vi "CatapultControl.vi"(10 "Fire Button":bool, 11 "ShooterDevRefIn":T1={"Wench Motor"={"DeviceStatus"={"status"=FALSE, "code"=0, "source"=""}, "Type"=enum."PWM", "PWM"={"Digital Module"=enum."Digital Module 1", "PWM Channel"=enum."Invalid", "DeadBand"={"Name"="", "maxPositivePwm"=0, "minPositivePwm"=0, "centerPwm"=0, "maxNegativePwm"=0, "minNegativePwm"=0, "angularRange"=0}}, "CAN"={"Device Number"=0, "Control Mode"=enum."Percent VBus", "Semaphore"=refnum, "Max Vout"=12.0}, "Invert"=FALSE, "TransformRef"=refnum, "InvTransformRef"=refnum}, "Lower Wench Limit"={"DevStatus"={"status"=FALSE, "code"=0, "source"=""}, "DIO Channel"=enum."DIO 1", "Digital Module"=enum."Digital Module 1"}, "Clutch Engaged Sensor"={"DevStatus"={"status"=FALSE, "code"=0, "source"=""}, "DIO Channel"=enum."DIO 1", "Digital Module"=enum."Digital Module 1"}, "Wench Encoder"={"DevStatus"={"status"=FALSE, "code"=0, "source"=""}, "EncoderIndex"=enum."Invalid", "CounterIndex"=enum."Invalid", "DistancePerCount"=1.0, "Decoding Type"=enum."4x"}, "Fire Sensor"={"DevStatus"={"status"=FALSE, "code"=0, "source"=""}, "DIO Channel"=enum."DIO 1", "Digital Module"=enum."Digital Module 1"}, "Worm Motor"={"DeviceStatus"={"status"=FALSE, "code"=0, "source"=""}, "Type"=enum."PWM", "PWM"={"Digital Module"=enum."Digital Module 1", "PWM Channel"=enum."Invalid", "DeadBand"={"Name"="", "maxPositivePwm"=0, "minPositivePwm"=0, "centerPwm"=0, "maxNegativePwm"=0, "minNegativePwm"=0, "angularRange"=0}}, "CAN"={"Device Number"=0, "Control Mode"=enum."Percent VBus", "Semaphore"=refnum, "Max Vout"=12.0}, "Invert"=FALSE, "TransformRef"=refnum, "InvTransformRef"=refnum}, "Minimum Worm Sensor"={"DevStatus"={"status"=FALSE, "code"=0, "source"=""}, "DIO Channel"=enum."DIO 1", "Digital Module"=enum."Digital Module 1"}, "Catapult Arm Pot"={"DevStatus"={"status"=FALSE, "code"=0, "source"=""}, "Analog Module"=enum."Analog Module 1", "Analog Channel"=enum."Invalid"}, "Forklift Pot"={"DevStatus"={"status"=FALSE, "code"=0, "source"=""}, "Analog Module"=enum."Analog Module 1", "Analog Channel"=enum."Invalid"}}) -> ()   [LabVIEW 2013]
uses:
  Utils/ShooterDevRef.ctl
  <vilib>/Rock Robotics/WPI/MotorControl/WPI_MotorControlDeviceRef.ctl
  <vilib>/Rock Robotics/SystemInterfaces/Typedef/FPGA_TypedefDigitalModule.ctl
  <vilib>/Rock Robotics/SystemInterfaces/DIO/FPGA_DIOPWMChannel.ctl
  <vilib>/Rock Robotics/WPI/PWM/WPI_PWMDeadband.ctl
  <vilib>/Rock Robotics/WPI/CAN/Jaguar/SubVIs/WPI_CANJaguar_ControlMode.ctl
  <vilib>/Rock Robotics/WPI/PWM/WPI_PWMTransform_ConPane.ctl
  <vilib>/Rock Robotics/WPI/DigitalInput/WPI_DigitalInputDevRef.ctl
  <vilib>/Rock Robotics/SystemInterfaces/DIO/FPGA_DIOChannel.ctl
  <vilib>/Rock Robotics/WPI/Encoder/WPI_EncoderDevRef.ctl
  <vilib>/Rock Robotics/SystemInterfaces/Encoder/FPGA_EncoderIdx.ctl
  <vilib>/Rock Robotics/SystemInterfaces/Counter/FPGA_CounterCtrSystemIndex.ctl
  <vilib>/Rock Robotics/WPI/Encoder/WPI_EncoderType.ctl
  <vilib>/Rock Robotics/WPI/AnalogChannel/WPI_AnalogChannelDevRef.ctl
  <vilib>/Rock Robotics/SystemInterfaces/Typedef/FPGA_TypedefAnalogModule.ctl
  <vilib>/Rock Robotics/SystemInterfaces/AI/FPGA_AIChannel.ctl
  Utils/ShooterStateEnum.ctl
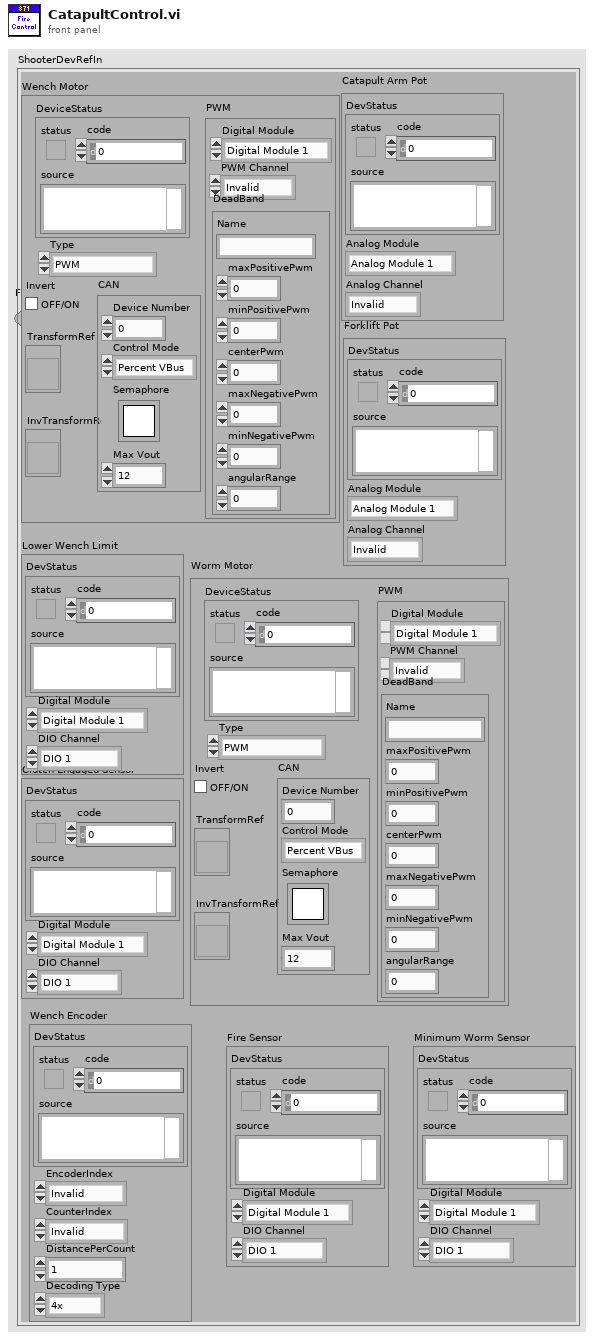
[diagram p1: front panel]
types:
  T1 = typedef "ShooterDevRef.ctl" = cluster{"Wench Motor":T2, "Lower Wench Limit":T9, "Clutch Engaged Sensor":T9, "Wench Encoder":T11, "Fire Sensor":T9, "Worm Motor":T2, "Minimum Worm Sensor":T9, "Catapult Arm Pot":T15, "Forklift Pot":T15}
  T2 = typedef "WPI_MotorControlDeviceRef.ctl" = cluster{"DeviceStatus":errorcluster, "Type":enum16{"PWM", "CAN"}, "PWM":cluster{"Digital Module":T3, "PWM Channel":T4, "DeadBand":T5}, "CAN":cluster{"Device Number":u8, "Control Mode":T6, "Semaphore":T7, "Max Vout":dbl}, "Invert":bool, "TransformRef":T8, "InvTransformRef":T8}
  T3 = typedef "FPGA_TypedefDigitalModule.ctl" = enum16{"Digital Module 1", "Digital Module 2"}
  T4 = typedef "FPGA_DIOPWMChannel.ctl" = enum8{"PWM 1", "PWM 2", "PWM 3", "PWM 4", "PWM 5", "PWM 6", "PWM 7", "PWM 8", "PWM 9", "PWM 10", "Invalid"}
  T5 = typedef "WPI_PWMDeadband.ctl" = cluster{"Name":string, "maxPositivePwm":i32, "minPositivePwm":i32, "centerPwm":i32, "maxNegativePwm":i32, "minNegativePwm":i32, "angularRange":u16}
  T6 = typedef "WPI_CANJaguar_ControlMode.ctl" = enum8{"Percent VBus", "Current", "Speed", "Position", "Voltage"}
  T7 = typedef "Semaphore RefNum" = refnum<k1>
  T8 = typedef "WPI_PWMTransform_ConPane.ctl" = refnum<vi>
  T9 = typedef "WPI_DigitalInputDevRef.ctl" = cluster{"DevStatus":errorcluster, "DIO Channel":T10, "Digital Module":T3}
  T10 = typedef "FPGA_DIOChannel.ctl" = enum8{"DIO 1", "DIO 2", "DIO 3", "DIO 4", "DIO 5", "DIO 6", "DIO 7", "DIO 8", "DIO 9", "DIO 10", "DIO 11", "DIO 12", "DIO 13", "DIO 14", "Invalid"}
  T11 = typedef "WPI_EncoderDevRef.ctl" = cluster{"DevStatus":errorcluster, "EncoderIndex":T12, "CounterIndex":T13, "DistancePerCount":dbl, "Decoding Type":T14}
  T12 = typedef "FPGA_EncoderIdx.ctl" = enum8{"Enc 0", "Enc 1", "Enc 2", "Enc 3", "Invalid"}
  T13 = typedef "FPGA_CounterCtrSystemIndex.ctl" = enum8{"Ctr 0", "Ctr 1", "Ctr 2", "Ctr 3", "Ctr 4", "Ctr 5", "Ctr 6", "Ctr 7", "Invalid"}
  T14 = typedef "WPI_EncoderType.ctl" = enum16{"1x", "2x", "4x"}
  T15 = typedef "WPI_AnalogChannelDevRef.ctl" = cluster{"DevStatus":errorcluster, "Analog Module":T16, "Analog Channel":T17}
  T16 = typedef "FPGA_TypedefAnalogModule.ctl" = enum16{"Analog Module 1", "Analog Module 2"}
  T17 = typedef "FPGA_AIChannel.ctl" = enum8{"AI 1", "AI 2", "AI 3", "AI 4", "AI 5", "AI 6", "AI 7", "AI 8", "Invalid"}
  T18 = typedef "ShooterStateEnum.ctl" = enum16{"Activate Clutch", "Engage Wench", "Stop Wench/ Wait for OP", "Disengage Clutch"}
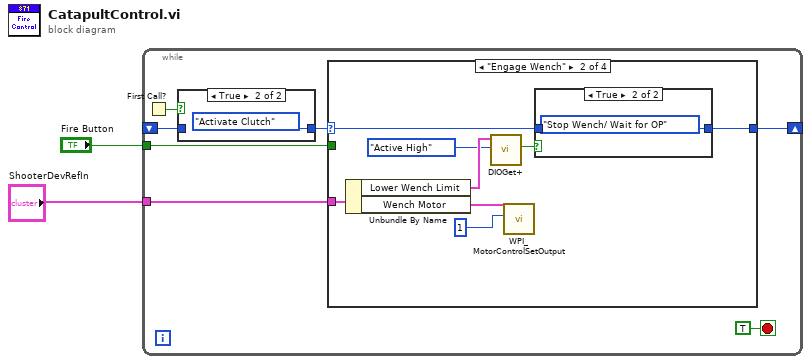
[diagram p0: block diagram]
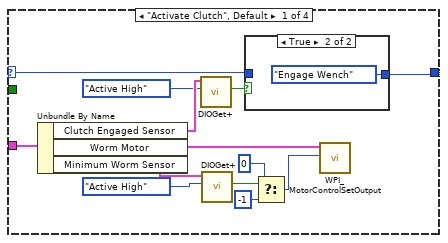
[diagram p3: hidden frame]
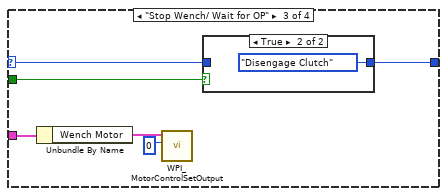
[diagram p6: hidden frame]
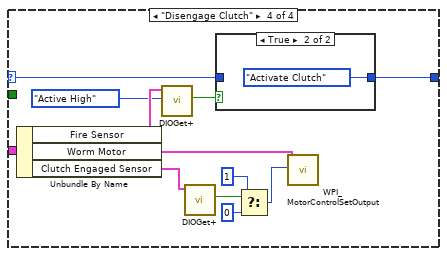
[diagram p8: hidden frame]
diagram:
  n1 = while {
    shift-right: [w6] -> _
    shift-left: _ -> [w7]
    tunnel: "ShooterDevRefIn" -> [w5]
    tunnel: "Fire Button" -> [w3]
    stop <- TRUE stop-if-true
    n2 = First Call?() -> (First Call?: T/F=w8:bool)
    n3 = case shown="True" w8 {
      tunnel: [w10 ShooterStateEnum."Activate Clutch" ("Enum")] -> w4
      tunnel: w7 -> [w10 _]
      frame False {
      }
      frame True {
      }
    }
    n4 = case shown="\"Engage Wench\"" w4 {
      selector: w4 -> [w19 w27 w37 w52]
      tunnel: [w20 w28 w38 w53] -> w6
      tunnel: w5 -> [w24 w34 w42 w56]
      tunnel: w3 -> [_ _ w39 _]
      frame "Activate Clutch", Default {
        n5 = Unbundle By Name(w24) -> ("Clutch Engaged Sensor"=w23:T9, "Worm Motor"=w18:T2, "Minimum Worm Sensor"=w17:T9)
        n6 = call "DIOGet+.vi"("Sensor Type"=enum16{"Active Low", "Active High"}."Active High", "DigitalInputDevRefIn"=w23) -> ("Value"=w22:bool)  [unwired: 7 in, 2 out]
        n7 = call "DIOGet+.vi"("Sensor Type"=enum16{"Active Low", "Active High"}."Active High", "DigitalInputDevRefIn"=w17) -> ("Value"=w15:bool)  [unwired: 7 in, 2 out]
        n8 = case shown="True" w22 {
          tunnel: [w25 ShooterStateEnum."Engage Wench" ("Enum")] -> w20
          tunnel: w19 -> [w25 _]
          frame False {
          }
          frame True {
          }
        }
        n9 = Select(t=0, s=w15, f=-1) -> (s? t:f=w12:i32)
        n10 = call <vilib>:"WPI_MotorControlSetOutput.vi"("Output"=w12, "MotorControlDevRef"=w18) -> ()  [unwired: 7 in, 3 out]
      }
      frame "Engage Wench" {
        n11 = Unbundle By Name(w34) -> ("Lower Wench Limit"=w31:T9, "Wench Motor"=w33:T2)
        n12 = call "DIOGet+.vi"("Sensor Type"=enum16{"Active Low", "Active High"}."Active High", "DigitalInputDevRefIn"=w31) -> ("Value"=w30:bool)  [unwired: 7 in, 2 out]
        n13 = call <vilib>:"WPI_MotorControlSetOutput.vi"("Output"=1, "MotorControlDevRef"=w33) -> ()  [unwired: 7 in, 3 out]
        n14 = case shown="True" w30 {
          tunnel: [w35 ShooterStateEnum."Stop Wench/ Wait for OP" ("Enum")] -> w28
          tunnel: w27 -> [w35 _]
          frame False {
          }
          frame True {
          }
        }
      }
      frame "Stop Wench/ Wait for OP" {
        n15 = Unbundle By Name(w42) -> ("Wench Motor"=w40:T2)
        n16 = call <vilib>:"WPI_MotorControlSetOutput.vi"("Output"=0, "MotorControlDevRef"=w40) -> ()  [unwired: 7 in, 3 out]
        n17 = case shown="True" w39 {
          tunnel: [w43 ShooterStateEnum."Disengage Clutch" ("Enum")] -> w38
          tunnel: w37 -> [w43 _]
          frame False {
          }
          frame True {
          }
        }
      }
      frame "Disengage Clutch" {
        n18 = Unbundle By Name(w56) -> ("Fire Sensor"=w55:T9, "Worm Motor"=w47:T2, "Clutch Engaged Sensor"=w45:T9)
        n19 = call "DIOGet+.vi"("Sensor Type"=enum16{"Active Low", "Active High"}."Active High", "DigitalInputDevRefIn"=w55) -> ("Value"=w54:bool)  [unwired: 7 in, 2 out]
        n20 = call "DIOGet+.vi"("DigitalInputDevRefIn"=w45) -> ("Value"=w50:bool)  [unwired: 8 in, 2 out]
        n21 = case shown="True" w54 {
          tunnel: [w57 ShooterStateEnum."Activate Clutch" ("Enum")] -> w53
          tunnel: w52 -> [w57 _]
          frame False {
          }
          frame True {
          }
        }
        n22 = Select(t=1, s=w50, f=0) -> (s? t:f=w46:i32)
        n23 = call <vilib>:"WPI_MotorControlSetOutput.vi"("Output"=w46, "MotorControlDevRef"=w47) -> ()  [unwired: 7 in, 3 out]
      }
    }
  }
